vi "Start Command.vi"(8 "error in":errorcluster, 11 "CIFCorePlugin in":refnum<class "CIFCorePlugin.lvclass">) -> (0 "error out":errorcluster, 3 "CIFCorePlugin out":refnum<class "CIFCorePlugin.lvclass">)   [LabVIEW 2021, in "CIFCorePlugin.lvclass"]
uses:
  CIFCorePlugin.lvclass
  Typedef/gRPC to Main Commands.ctl
  0124de93-67bc-4437-967e-5a501b30d5f0.vi
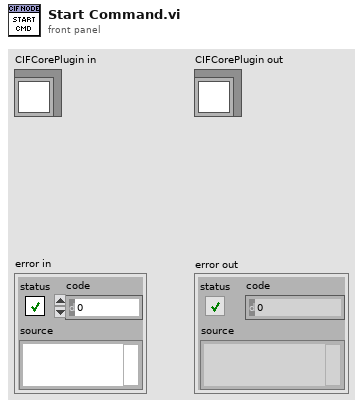
[diagram p1: front panel]
types:
  T1 = typedef "CIFCorePlugin.lvclass/gRPC to Main Commands.ctl" = enum8{"Start", "Pause", "Stop", "RefreshStats", "UpdateConfig", "Update Clock Map", "Connect Channel", "Force Channel", "Add Publisher Instance", "Remove Publisher Instance"}
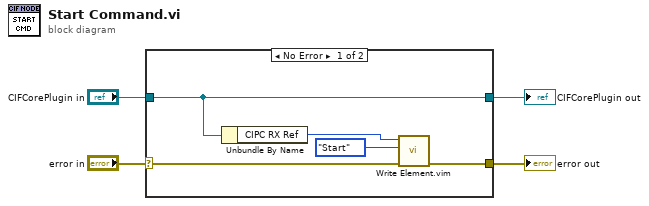
[diagram p0: block diagram]
diagram:
  n1 = case shown="No Error" "error in" {
    selector: "error in" -> [w9 w11]
    tunnel: [w7 w11] -> w3
    tunnel: "CIFCorePlugin in" -> [w5 w10]
    tunnel: [w5 w10] -> w1
    frame No Error {
      n2 = Unbundle By Name(w5) -> ("CIPC RX Ref"=w6:u64)
      n3 = call "Write Element.vim"("error in (no error)"=w9, "Data in"=gRPC_to_Main_Commands."Start" ("OOB Main Commands"), "CIPC Reference in"=w6) -> ("error out"=w7:errorcluster)  [unwired: 5 in, 3 out]
    }
    frame Error {
    }
  }
  "error out" <- w3
  "CIFCorePlugin out" <- w1
